vi "Test Call Global Teardown.vi"(8 "error in (no error)":errorcluster, 11 "Test Case In":refnum<class "Global Fixture Test.lvclass">) -> (0 "error out":errorcluster, 3 "Test Case Out":refnum<class "Global Fixture Test.lvclass">)   [LabVIEW 2020, in "Global Fixture Test.lvclass"]
uses:
  Global Fixture Test.lvclass
  C:/Program Files (x86)/National Instruments/LabVIEW 2020/vi.lib/Astemes/LUnit/Test Case.lvclass
  source/Global Fixture Test Double/Global Fixture Test Double.lvclass
  <vilib>/Astemes/LUnit/Test Case.lvclass/Test Case.ctl
  eb2f74be-2371-49fc-b197-683e86c0698c.vi
  <vilib>/Astemes/LUnit/Append Pass Result.vi
  <vilib>/Astemes/LUnit/Append Fail Result.vi
  <vilib>/Astemes/LUnit/Describe Comparison.vi
  <vilib>/Astemes/LUnit/Compare Variants.vi
  <vilib>/Astemes/LUnit/Test Suite.lvclass
  C:/Program Files (x86)/National Instruments/LabVIEW 2020/vi.lib/Astemes/LUnit/LUnit Runnable.lvclass
  <vilib>/Astemes/LUnit/Describe Variant.vi
  <vilib>/Astemes/LUnit/LUnit Runnable.lvclass
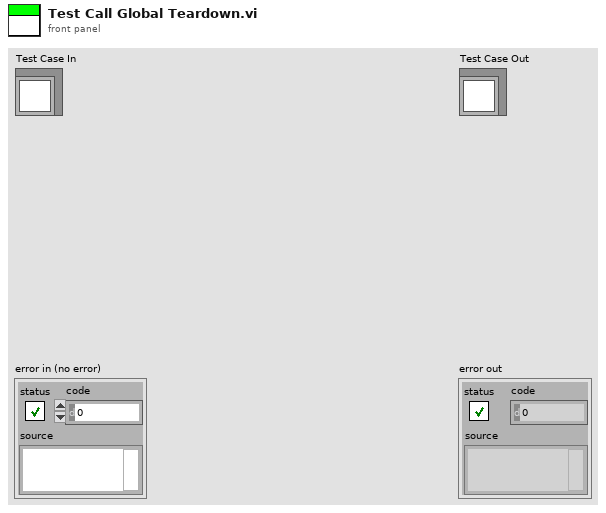
[diagram p1: front panel]
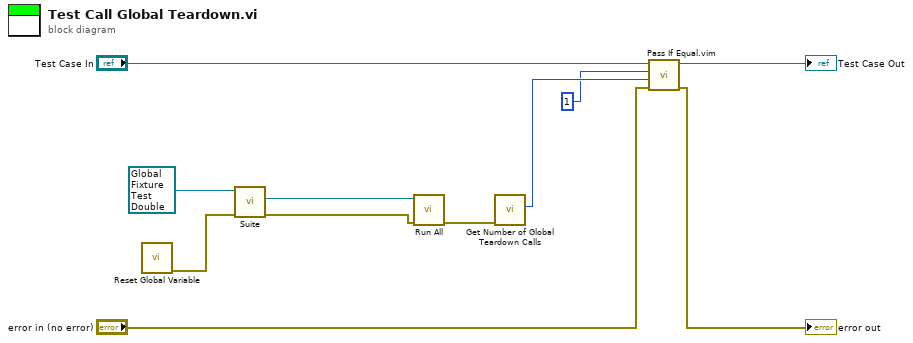
[diagram p0: block diagram]
diagram:
  n1 = call "Reset Global Variable.vi"() -> ("error out"=w7:errorcluster)  [unwired: 11 in]
  n2 = call-dynamic "Suite.vi"("error in (no error)"=w7, "Global Fixture Test Case Class in"=refnum<class "Global Fixture Test Double.lvclass"> refnum ("Global Fixture Test Double.lvclass")) -> ("error out"=w1:errorcluster, "LUnit Test Suite Out"=w3:refnum<class "Test Suite.lvclass">)  [unwired: 7 in, 1 out]
  n3 = call <vilib>:"Run All.vi"("error in (no error)"=w1, "Runnable In"=w3) -> ("error out"=w2:errorcluster)  [unwired: 8 in, 1 out]
  n4 = call "Get Number of Global Teardown Calls.vi"("error in (no error)"=w2) -> ("Calls to Teardown"=w5:i32)  [unwired: 9 in, 1 out]
  n5 = call "Pass If Equal.vim"("error in (no error)"="error in (no error)", "Actual"=w5, "Expected"=1 ("Calls to Setup"), "LUnit Test Case In"="Test Case In") -> ("error out"=→"error out":errorcluster, "LUnit Test Case Out"=→"Test Case Out":refnum<class "Global Fixture Test.lvclass">)  [unwired: 6 in]
